vi "StartTrial.vi"(8 "error in (no error)":errorcluster, 11 "TrialBasedExperiment in":refnum<class "FleTraining.lvclass">=refnum) -> (0 "error out":errorcluster, 3 "TrialBasedExperiment out":refnum<class "FleTraining.lvclass">)   [LabVIEW 2014, in "FleTraining.lvclass"]
uses:
  FleTraining.lvclass
  Acquisition/BehaviorData/BehaviorData.lvclass
  FleTraining.lvclass/FleTraining.ctl
  TwoAfcEye/TwoAfcEye.lvclass
  Matlab API/Matlab API.lvlib
panel:
  in  "expMode":bool=TRUE
  in  "trajectoryLength":dbl=1600.0
  in  "randReward":bool
  in  "maxBlockSize":dbl=2.0
  in  "randLocation":bool
  in  "relDelayTime":dbl=200.0
  in  "noFlashZone":dbl=100.0
  in  "flashLocation":dbl=500.0
  in  "perceivedLag":dbl
  in  "yOffset":dbl=336.0
  in  "flashOffset":dbl=250.0
  in  "flashDuration":dbl=1.0
  in  "speed":dbl=1359.0
  in  "trajectoryAngle":dbl
  in  "trajectoryCenterY":dbl=506.0
  in  "trajectoryCenterX":dbl=800.0
  in  "condRepeatType":string(combo)="None"
  in  "punishType":string(combo)="IncorrRespAndAborts"
  in  "punishTime":dbl
  in  "playResponseSounds":bool
  in  "targetRadius":dbl=100.0
  in  "lagProb":dbl(slide)=0.5 scale=0.0..1.0
  in  "moveProb":dbl(slide)=0.5 scale=0.0..1.0
  # "If expMode is switched on\nflash offsets and locations are\ntaken from the configuration file \ninstead of the front panel."
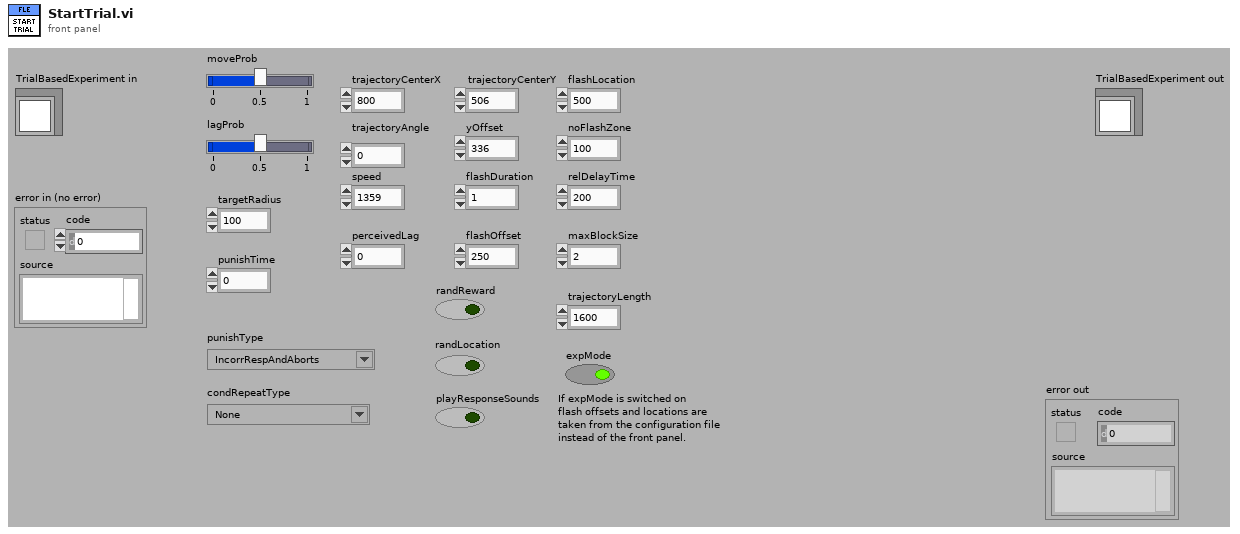
[diagram p1: front panel]
types:
  T1 = cluster{"Intertrial":dbl, "AcquireFixation":dbl, "HoldFixation":dbl, "DelayPeriod":dbl, "ResponsePeriod":dbl}
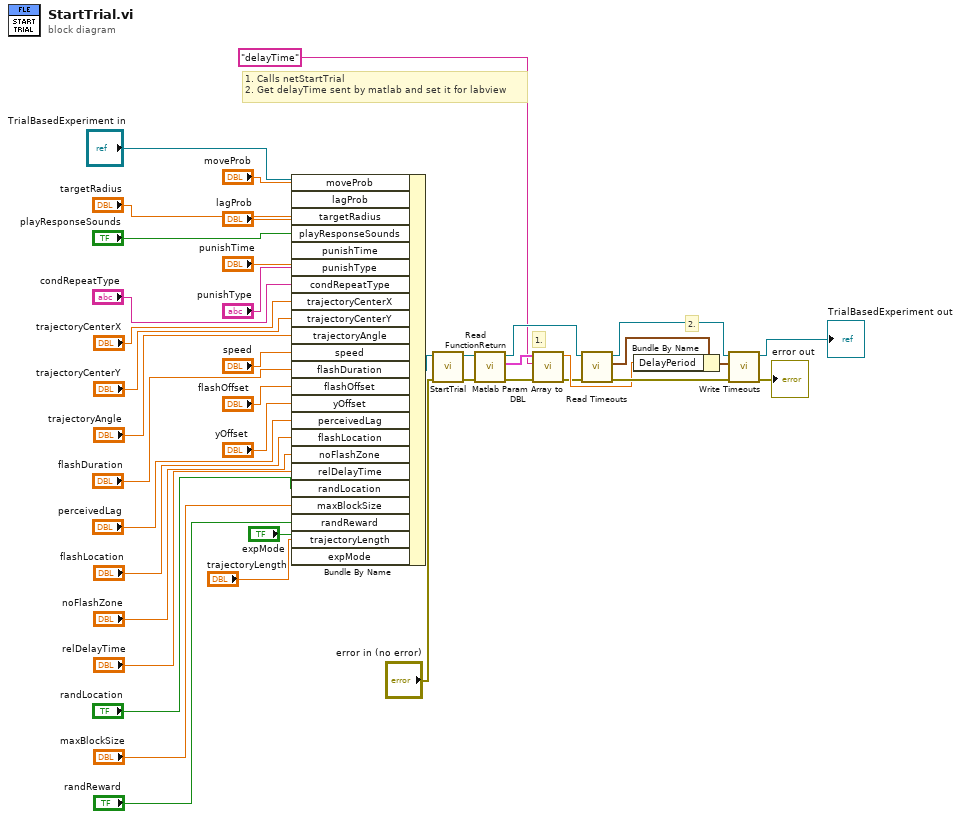
[diagram p0: block diagram]
diagram:
  # "1. Calls netStartTrial\n2. Get delayTime sent by matlab and set it for labview"
  # "2."
  # "1."
  n1 = Bundle By Name(cluster="TrialBasedExperiment in", "moveProb"="moveProb", "lagProb"="lagProb", "targetRadius"="targetRadius", "playResponseSounds"="playResponseSounds", "punishTime"="punishTime", "punishType"="punishType", "condRepeatType"="condRepeatType", "trajectoryCenterX"="trajectoryCenterX", "trajectoryCenterY"="trajectoryCenterY", "trajectoryAngle"="trajectoryAngle", "speed"="speed", "flashDuration"="flashDuration", "flashOffset"="flashOffset", "yOffset"="yOffset", "perceivedLag"="perceivedLag", "flashLocation"="flashLocation", "noFlashZone"="noFlashZone", "relDelayTime"="relDelayTime", "randLocation"="randLocation", "maxBlockSize"="maxBlockSize", "randReward"="randReward", "trajectoryLength"="trajectoryLength", "expMode"="expMode") -> (w24:refnum<class "FleTraining.lvclass">)
  n2 = call-parent "StartTrial.vi"("error in (no error)"="error in (no error)", "TrialBasedExperiment in"=w24) -> ("error out"=w30:errorcluster, "TrialBasedExperiment out"=w27:refnum<class "FleTraining.lvclass">)  [unwired: 8 in]
  n3 = call-dynamic "Read FunctionReturn.vi"("error in (no error)"=w30, "MatlabExperiment in"=w27) -> ("error out"=w32:errorcluster, "FunctionReturn"=w37:cluster{"Name":string, "Data":variant}[], "MatlabExperiment out"=w40:refnum<class "FleTraining.lvclass">)  [unwired: 7 in]
  n4 = call "Matlab Param Array to DBL.vi"("error in (no error)"=w32, "Name"="delayTime", "Matlab Param Array"=w37) -> ("error out"=w31:errorcluster, "data"=w34:dbl)  [unwired: 7 in]
  n5 = call-dynamic "Read Timeouts.vi"("error in (no error)"=w31, "TrialBasedExperiment in"=w40) -> ("error out"=w38:errorcluster, "Timeouts"=w35:T1, "TrialBasedExperiment out"=w39:refnum<class "FleTraining.lvclass">)  [unwired: 7 in]
  n6 = Bundle By Name(cluster=w35, "DelayPeriod"=w34) -> (w33:T1)
  n7 = call-dynamic "Write Timeouts.vi"("error in (no error)"=w38, "Timeouts"=w33, "TrialBasedExperiment in"=w39) -> ("error out"=→"error out":errorcluster, "TrialBasedExperiment out"=→"TrialBasedExperiment out":refnum<class "FleTraining.lvclass">)  [unwired: 7 in]
